vi "Read VI Data File.vi"(8 "error in":errorcluster, 11 "Path":path) -> (0 "error out":errorcluster, 1 "Type":T1[](array[typedef]), 2 "Data":variant[](array[variant]))   [LabVIEW 2019]
doc: "Drop this VI into any VI will save a copy of the data on the front panel as a VI without a diagram."
uses:
  <vilib>/Utility/Data Type/Type Definitions/Data Type.ctl
  <vilib>/Utility/Data Type/NI_Data Type.lvlib
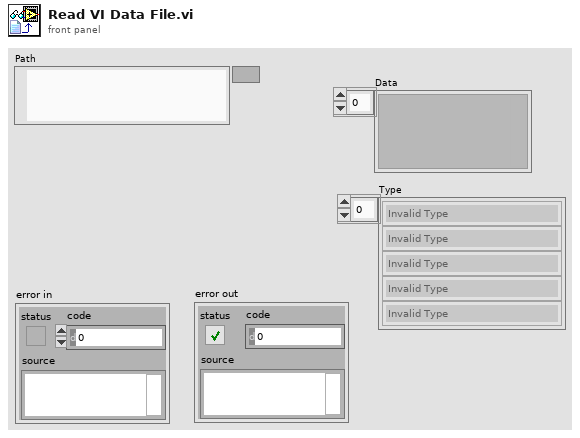
[diagram p1: front panel]
types:
  T1 = typedef "NI_Data Type.lvlib/Data Type.ctl" = enum8{"Invalid Type", "Void", "I8", "I16", "I32", "I64", "U8", "U16", "U32", "U64", "Single Float", "Double Float", "Extended Float", "Single Complex", "Double Complex", "Extended Complex", "Enum U8", "Enum U16", "Enum U32", "Enum U64", "Single Float With Unit", "Double Float With Unit", "Extended Float With Unit", "Single Complex with Unit", "Double Complex with Unit", "Extended Complex with Unit", "Boolean", "String", "Path", "Picture", "Tag", "Array", "Cluster", "Variant", "LV Variant", "Waveform", "Timestamp", "Digital Waveform", "Digital Data", "ExpressData", "Refnum", "External Data", "VI", "Poly VI", "LabVIEW Class Instance", "Fixed Point", "Set Collection", "Map Collection"}
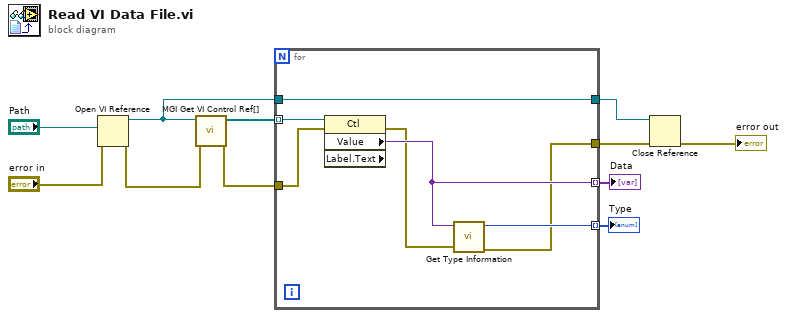
[diagram p0: block diagram]
diagram:
  n1 = Open VI Reference(vi path="Path", error in (no error)="error in") -> (vi reference=w5:refnum<vi>, error out=w10:errorcluster)  [unwired: 4 in]
  n2 = call <userlib>:"MGI Get VI Control Ref[].vi"("error in"=w10, "VI (Caller)"=w5) -> ("error out"=w4:errorcluster, "Control[i]"=w9:refnum<vi>[])  [unwired: 6 in, 2 out]
  n3 = for {
    tunnel: w9 -> [w18] mode=indexing
    tunnel: w4 -> [w17]
    tunnel: [w12] -> w8
    tunnel: [w16] -> w7
    tunnel: w5 -> [w16]
    tunnel: [w15] -> w2 mode=indexing
    tunnel: [w14] -> w1 mode=indexing
    n4 = property class="Ctl" props=["Value", "Label", "Text"](reference=w18, error in=w17) -> (error out=w13:errorcluster, "Value"=w15:variant)  [unwired: 2 out]
    n5 = call <vilib>:"Get Type Information.vi"("error in (no error)"=w13, "variant"=w15) -> ("error out"=w12:errorcluster, "type"=w14:T1)  [unwired: 5 in, 3 out]
  }
  "Data" <- w2
  "Type" <- w1
  n6 = Close Reference(reference=w7, error in (no error)=w8) -> (error out=→"error out":errorcluster)
